vi "In16ToIn32CDAB.vi"(8 "error in (no error)":errorcluster, 9 "length":i32=15, 10 "index":i32, 11 "Input Registers":u16[](array[numeric])) -> (0 "error out":errorcluster, 3 "Output Registers":i32[](array[numeric]))   [LabVIEW 2016]
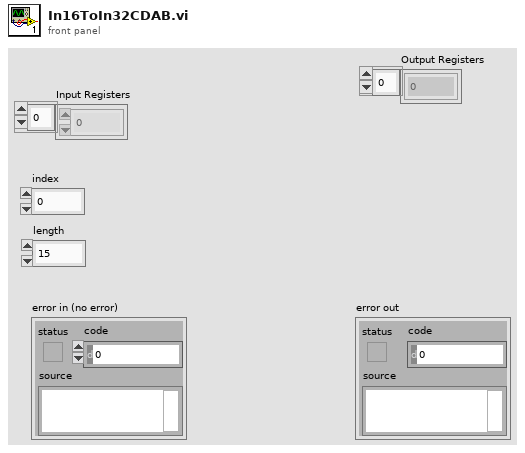
[diagram p1: front panel]
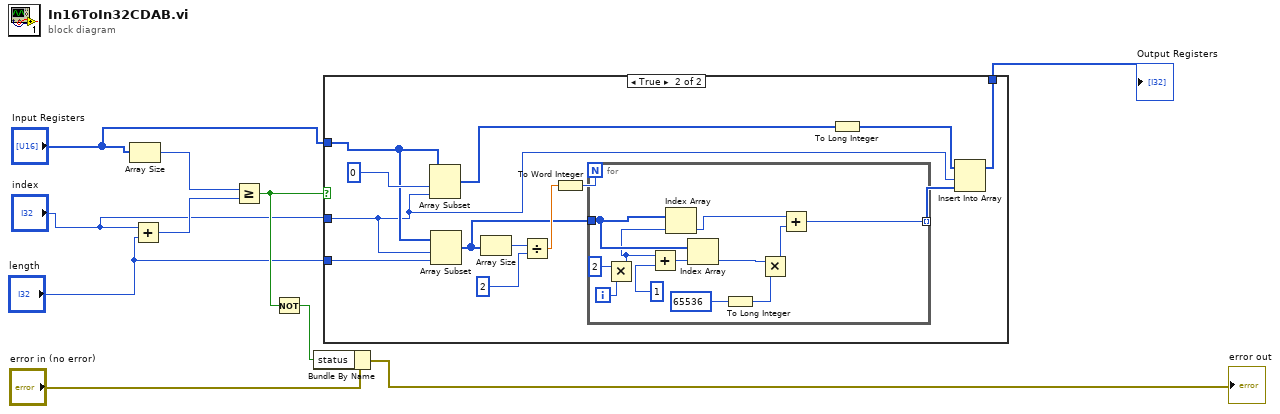
[diagram p0: block diagram]
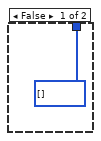
[diagram p2: hidden frame]
diagram:
  n1 = Array Size(array="Input Registers") -> (size(s)=w10:i32)
  n2 = Add(x="index", y="length") -> (x+y=w9:i32)
  n3 = Greater Or Equal?(x=w10, y=w9) -> (x >= y?=w8:bool)
  n4 = Not(x=w8) -> (.not. x?=w5:bool)
  n5 = Bundle By Name(cluster="error in (no error)", "status"=w5) -> (→"error out":errorcluster)
  n6 = case shown="True" w8 {
    tunnel: "Input Registers" -> [_ w23]
    tunnel: "index" -> [_ w15]
    tunnel: "length" -> [_ w22]
    tunnel: [u16[] [] w14] -> w1
    frame False {
    }
    frame True {
      n7 = Array Subset(array=w23, index=0, length=w15) -> (w13:u16[])
      n8 = Array Subset(array=w23, index=w15, length=w22) -> (w17:u16[])
      n9 = Array Size(array=w17) -> (size(s)=w21:i32)
      n10 = Divide(x=w21, y=2) -> (x/y=w18:dbl)
      n11 = To Word Integer(number=w18) -> (16bit integer=w19:i16)
      n12 = for {
        N: w19 -> [_]
        tunnel: w17 -> [w36]
        tunnel: [w30] -> w16 mode=indexing
        i -> [w28]
        n13 = Multiply(x=2, y=w28) -> (x*y=w26:i32)
        n14 = Add(x=w26, y=1) -> (x+y=w35:i32)
        n15 = Index Array(array=w36, index=w26) -> (element=w32:u16)
        n16 = Index Array(array=w36, index=w35) -> (element=w33:u16)
        n17 = To Long Integer(number=65536) -> (32bit integer=w29:i32)
        n18 = Multiply(x=w33, y=w29) -> (x*y=w31:i32)
        n19 = Add(x=w32, y=w31) -> (x+y=w30:i32)
      }
      n20 = To Long Integer(number=w13) -> (32bit integer=w12:i32[])
      n21 = Insert Into Array(array=w12, index=w15, new element=w16) -> (w14:i32[])
    }
  }
  "Output Registers" <- w1
